vi "Auto Deskew Process.vi"(8 "error in (no error)":errorcluster, 11 "VISA resource name":refnum<visa-resource-name>) -> (0 "error out":errorcluster, 3 "VISA resource name out":refnum<visa-resource-name>)   [LabVIEW 2016, in "Agilent 2000 3000 X-Series.lvlib"]
doc: "Launches the auto deskew process on the oscilloscope.\n\n<B>Note(s):</B>\nBefore run this VI:\n1. Demagnetize and zero- adjust the current probe.\nRefer to the current probe's documentation for instructions on how to do this.\n\n2. Make connections to the U1880A deskew fixture as described in the oscilloscope's connection dialog or in the DSOX3PWR Power Measurement Application User's Guide.\n\n3. Make sure the voltage probe and current probe channels are specified appropriately using Configure Power Signals Source.vi."
uses:
  Agilent 2000 3000 X-Series.lvlib
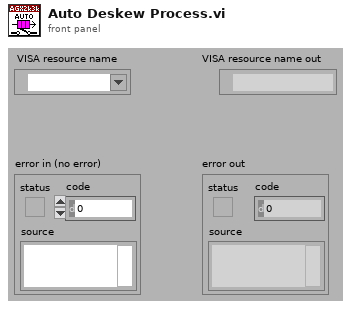
[diagram p1: front panel]
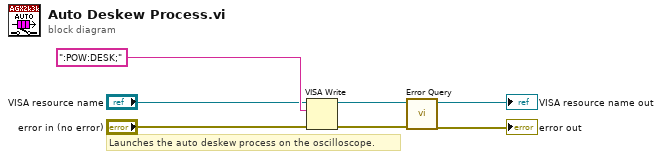
[diagram p0: block diagram]
diagram:
  # "Launches the auto deskew process on the oscilloscope."
  n1 = VISA Write(VISA resource name="VISA resource name", write buffer=":POW:DESK;", error in (no error)="error in (no error)") -> (VISA resource name out=w4:refnum<visa-resource-name>, error out=w3:errorcluster)  [unwired: 1 out]
  n2 = call "Error Query.vi"("error in (no error)"=w3, "VISA resource name"=w4) -> ("error out"=→"error out":errorcluster, "VISA resource name out"=→"VISA resource name out":refnum<visa-resource-name>)  [unwired: 8 out]
